vi "Error Query.vi"(8 "error in (no error)":errorcluster, 11 "VISA resource name":refnum<visa-resource-name>) -> (0 "error out":errorcluster, 1 "Error Message":string, 2 "Error Code":i32[](array[numeric]), 3 "VISA resource name out":refnum<visa-resource-name>)   [LabVIEW 2025, in "Chroma 19572.lvlib"]
doc: "Queries the instrument for any errors in the instrument's error queue. It will continue to read errors until all errors have been read from the instrument. Any errors will be returned in the <B>error out</B> control.\n\n<B>Note:</B>\nThis VI is called automatically by most driver VIs so it is not usually necessary to call this in an application."
uses:
  <instrlib>/Chroma 19572/Chroma 19572.lvlib
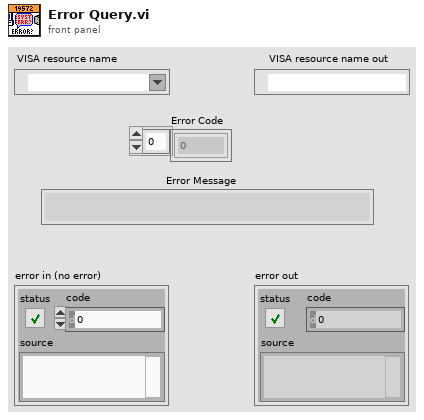
[diagram p1: front panel]
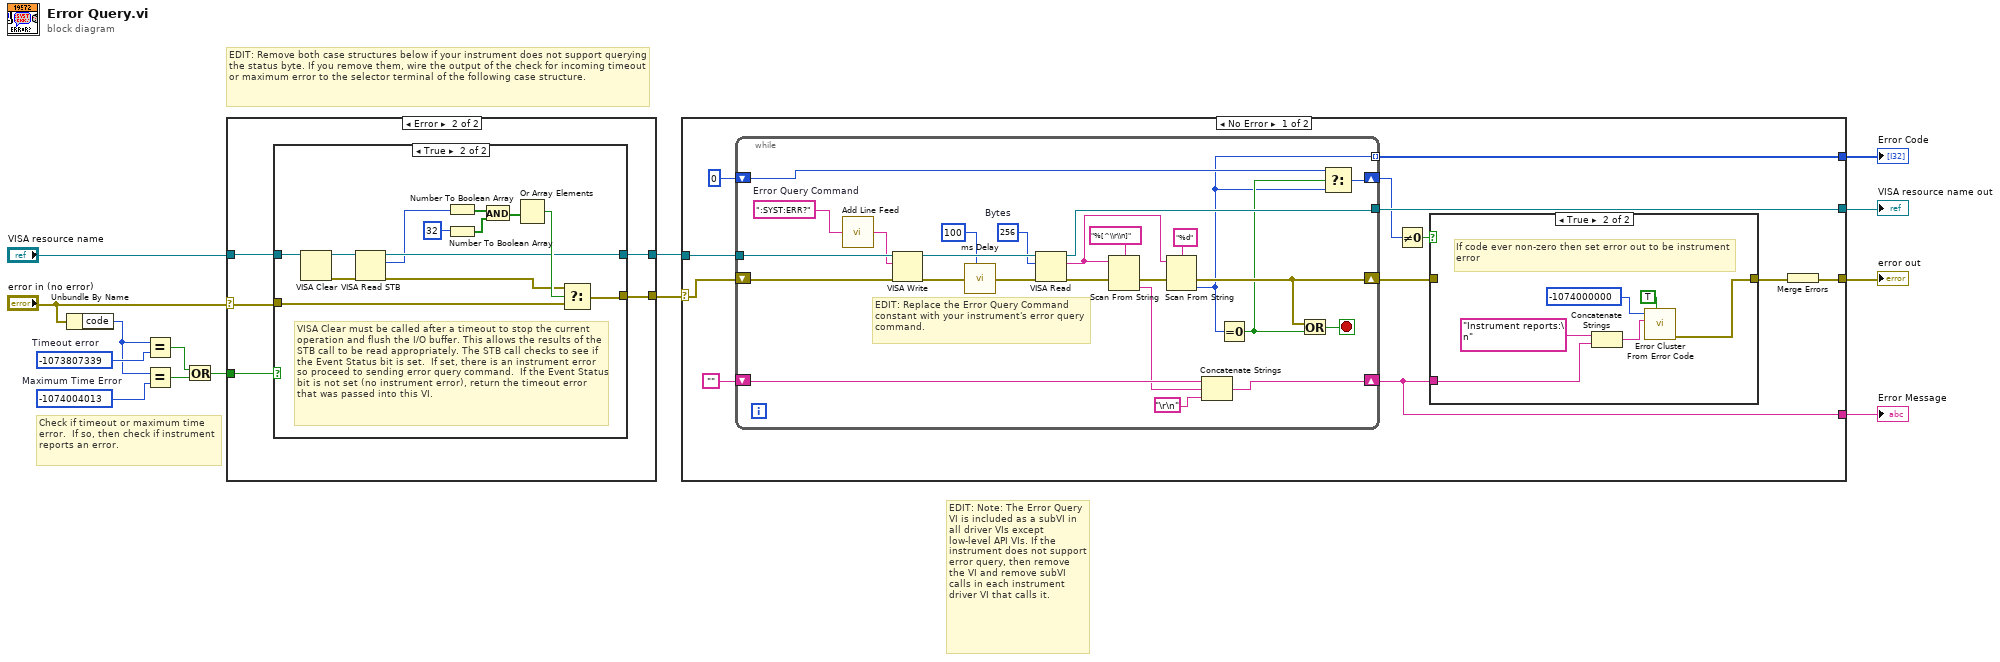
[diagram p0: block diagram]
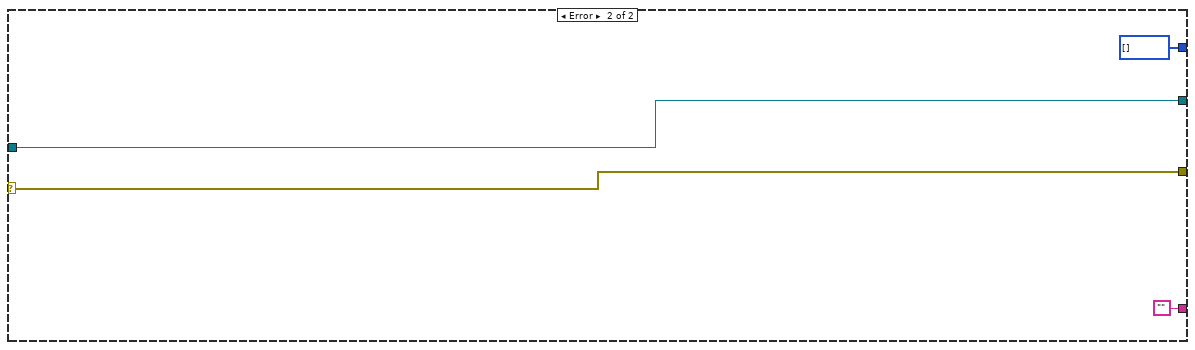
[diagram p5: hidden frame]
diagram:
  w7 = -1074004013  # Maximum Time Error
  w9 = -1073807339  # Timeout error
  # "EDIT: Note: The Error Query VI is included as a subVI in all driver VIs except low-level API VIs. If the instrument does not support error query, then remove the VI and remove subVI calls in each instrument driver VI that calls it."
  # "Check if timeout or maximum time error.  If so, then check if instrument reports an error."
  # "EDIT: Remove both case structures below if your instrument does not support querying the status byte. If you remove them, wire the output of the check for incoming timeout or maximum error to the selector terminal of the following case structure."
  n1 = Unbundle By Name("error in (no error)") -> ("code"=w8:i32)
  n2 = Equal?(x=w8, y=w9) -> (x = y?=w5:bool)
  n3 = Equal?(x=w8, y=w7) -> (x = y?=w6:bool)
  n4 = Or(x=w5, y=w6) -> (x .or. y?=w4:bool)
  n5 = case shown="Error" "error in (no error)" {
    selector: "error in (no error)" -> [w15 w19]
    tunnel: "VISA resource name" -> [w16 w21]
    tunnel: [w16 w20] -> w11
    tunnel: [w15 w18] -> w12
    tunnel: w4 -> [_ w17]
    frame No Error {
    }
    frame Error {
      n6 = case shown="True" w17 {
        tunnel: w21 -> [w23 w29]
        tunnel: [w23 w26] -> w20
        tunnel: w19 -> [w22 w32]
        tunnel: [w22 w31] -> w18
        frame False {
          # "Error code not a timeout, so best to pass on to user."
        }
        frame True {
          # "VISA Clear must be called after a timeout to stop the current operation and flush the I/O buffer. This allows the results of the  STB call to be read appropriately. The STB call checks to see if the Event Status bit is set.  If set, there is an instrument error so proceed to sending error query command.  If the Event Status bit is not set (no instrument error), return the timeout error that was passed into this VI."
          n7 = VISA Clear(VISA resource name=w29) -> (VISA resource name out=w28:refnum<visa-resource-name>, error out=w27:errorcluster)  [unwired: 1 in]
          n8 = VISA Read STB(8:w27, 11:w28) -> (0:w25:errorcluster, 2:w24:u16, 3:w26:refnum<visa-resource-name>)
          n9 = Number To Boolean Array(number=w24) -> (Boolean array=w33:bool[])
          n10 = Number To Boolean Array(number=32) -> (Boolean array=w35:bool[])
          n11 = And(x=w33, y=w35) -> (x .and. y?=w34:bool[])
          n12 = Or Array Elements(Boolean array=w34) -> (logical OR=w30:bool)
          n13 = Select(t=w25, s=w30, f=w32) -> (s? t:f=w31:errorcluster)
        }
      }
    }
  }
  n14 = case shown="No Error" w12 {
    selector: w12 -> [w37 w81]
    tunnel: [w48 w84] -> w2
    tunnel: w11 -> [w47 w84]
    tunnel: [w45 w81] -> w1
    tunnel: [w40 ""] -> w14
    tunnel: [w39 i32[] []] -> w13
    frame No Error {
      n15 = while {
        tunnel: [w79] -> w48
        tunnel: w47 -> [w78]
        shift-right: [w68] -> w40
        shift-left: "" -> [w71]
        shift-right: [w66] -> w41
        shift-left: 0 -> [w67]
        shift-right: [w80] -> w38
        shift-left: w37 -> [w65]
        tunnel: [w61] -> w39 mode=indexing
        stop <- w74 stop-if-true
        w76 = u32 256  # Bytes
        w60 = ":SYST:ERR?"  # Error Query Command
        # "EDIT: Replace the Error Query Command constant with your instrument's error query command."
        n16 = call <instrlib>:"Add Line Feed.vi"("Command string"=w60) -> ("Concatenated string"=w59:string)  [unwired: 4 in]
        n17 = VISA Write(VISA resource name=w78, write buffer=w59, error in (no error)=w65) -> (VISA resource name out=w77:refnum<visa-resource-name>, error out=w57:errorcluster)  [unwired: 1 out]
        n18 = call <instrlib>:"ms Delay.vi"("miliseconds to wait"=u32 100, "error in (no error)"=w57) -> ("error out"=w56:errorcluster)  [unwired: 6 in, 1 out]
        n19 = VISA Read(VISA resource name=w77, byte count=w76, error in (no error)=w56) -> (VISA resource name out=w79:refnum<visa-resource-name>, read buffer=w72:string, error out=w64:errorcluster)  [unwired: 1 out]
        n20 = Scan From String(format string="%[^\\r\\n]", input string=w72, error in=w64) -> (error out=w63:errorcluster, output 1=w69:string)  [unwired: 2 in, 2 out]
        n21 = Scan From String(format string="%d", input string=w72, error in=w63) -> (error out=w80:errorcluster, output 1=w61:i32)  [unwired: 2 in, 2 out]
        n22 = Concatenate Strings(w71, w69, "\r\n") -> (w68:string)
        n23 = Equal To 0?(x=w61) -> (x = 0?=w62:bool)
        n24 = Or(x=w80, y=w62) -> (x .or. y?=w74:bool)
        n25 = Select(t=w67, s=w62, f=w61) -> (s? t:f=w66:i32)
      }
      n26 = Not Equal To 0?(x=w41) -> (x != 0?=w43:bool)
      n27 = case shown="True" w43 {
        tunnel: w40 -> [_ w50]
        tunnel: [w49 w51] -> w42
        tunnel: w38 -> [w49 _]
        frame False {
        }
        frame True {
          # "If code ever non-zero then set error out to be instrument error"
          n28 = Concatenate Strings("Instrument reports:\n" ("Source"), w50) -> (w52:string)
          n29 = call <vilib>:"Error Cluster From Error Code.vi"("show call chain? (False)"=TRUE, "error message (\"\")"=w52, "error code (0)"=-1074000000 ("Code")) -> ("error out"=w51:errorcluster)  [unwired: 6 in]
        }
      }
      n30 = Merge Errors(w42) -> (w45:errorcluster)
    }
    frame Error {
    }
  }
  "Error Message" <- w14
  "Error Code" <- w13
  "VISA resource name out" <- w2
  "error out" <- w1
